vi "Input 信息检测.vi"(9 "Input 配置信息":string[][](table)=[["名称", "点位", "索引号", "逻辑取反"], ["启动按钮", "X100", "0", "0"], ["复位按钮", "X101", "1", "0"], ["暂停按钮", "X102", "2", "0"], ["操作侧安全光栅", "X103", "3", "0"], ["后侧安全光栅", "X104", "4", "0"], ["上层真空检知", "X105", "5", "0"], ["下层真空检知", "X106", "6", "0"], ["上层感应sensor", "X107", "7", "0"], ["下层感应sensor", "X110", "8", "0"], ["传送抓手气缸前位", "X111", "9", "0"], ["传送抓手气缸后位", "X112", "10", "0"], ["上层产品定位气缸前位", "X113", "11", "0"], ["上层产品定位气缸后位", "X114", "12", "0"], ["下层产品定位气缸前位", "X115", "13", "0"], ["下层产品定位气缸后位", "X116", "14", "0"], ["抓手感应产品sensor", "X117", "15", "0"], ["起子1真空检知", "X120", "16", "0"], ["起子2真空检知", "X121", "17", "0"], ["起子3真空检知", "X122", "18", "0"], ["起子4真空检知", "X123", "19", "0"], ["feed01感应sensor", "X124", "20", "0"], ["feed02感应sensor", "X125", "21", "0"], ["feed03感应sensor", "X126", "22", "0"], ["feed04感应sensor", "X127", "23", "0"], ["动子1和2统一坐标sensor", "X130", "24", "0"], ["动子3和4统一坐标sensor", "X131", "25", "0"], ["前后侧统一坐标sensor", "X132", "26", "0"], ["上站允许取料信号", "X133", "27", "0"], ["下站允许投料信号", "X134", "28", "0"], ["上站请求信号", "X135", "29", "0"], ["下站答复信号", "X136", "30", "0"]], 11 "输入":T1) -> (2 "Input  ERROR":string[](array[string]))   [LabVIEW 2017]
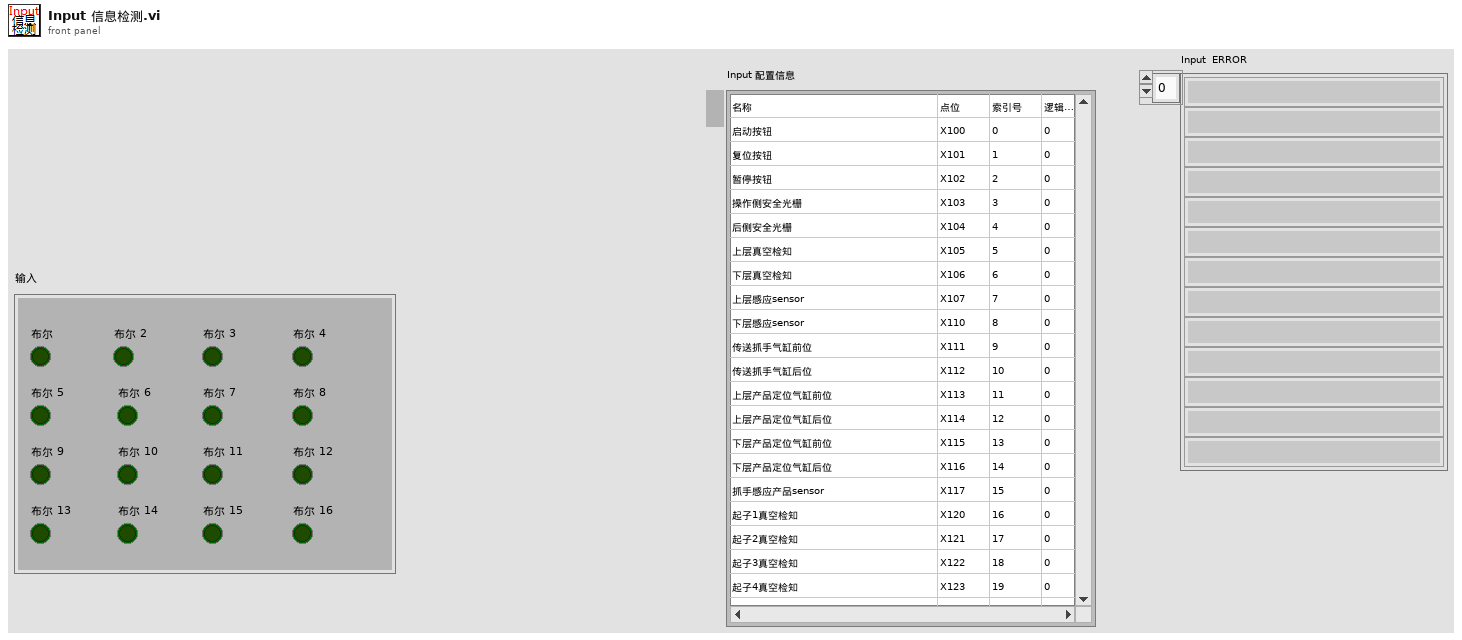
[diagram p1: front panel]
types:
  T1 = typedef "input控件.ctl" = cluster{"布尔":bool, "布尔 2":bool, "布尔 3":bool, "布尔 4":bool, "布尔 5":bool, "布尔 6":bool, "布尔 7":bool, "布尔 8":bool, "布尔 9":bool, "布尔 10":bool, "布尔 11":bool, "布尔 12":bool, "布尔 13":bool, "布尔 14":bool, "布尔 15":bool, "布尔 16":bool}
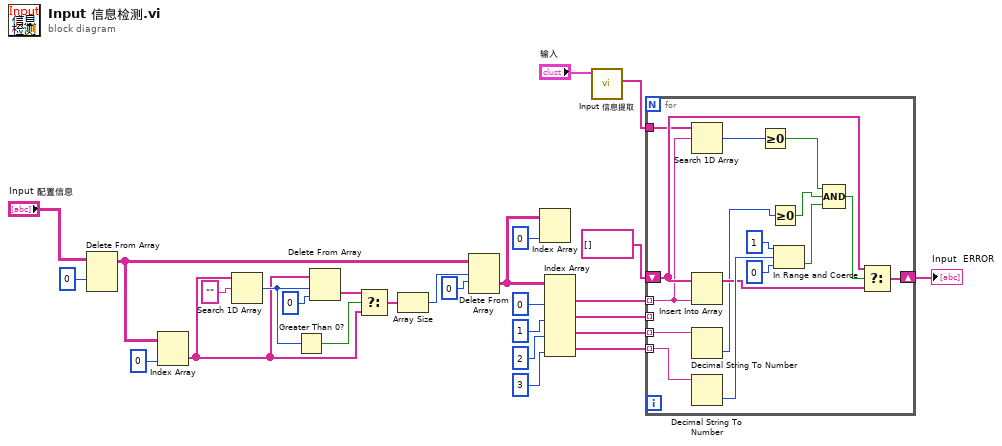
[diagram p0: block diagram]
diagram:
  n1 = Delete From Array(array="Input 配置信息", index (row)=0 ("索引 (行)")) -> (array with subset deleted=w13:string[][])  [unwired: 2 in, 1 out]
  n2 = Index Array(array=w13, index (col)=0 ("禁用的索引 (列)")) -> (element=w16:string[])  [unwired: 1 in]
  n3 = Search 1D Array(1D array=w16, element="") -> (index of element=w20:i32)  [unwired: 1 in]
  n4 = Greater Than 0?(x=w20) -> (x > 0?=w21:bool)
  n5 = Delete From Array(array=w16, length=w20, index=0 ("索引")) -> (deleted portion=w18:string[])  [unwired: 1 out]
  n6 = Select(t=w18, s=w21, f=w16) -> (s? t:f=w15:string[])
  n7 = Array Size(array=w15) -> (size(s)=w17:i32)
  n8 = Delete From Array(array=w13, length=w17, index (row)=0 ("索引 (行)")) -> (deleted portion=w2:string[][])  [unwired: 1 in, 1 out]
  n9 = Index Array(array=w2, index (col)=0 ("禁用的索引 (列)")) -> ()  [unwired: 1 in, 1 out]
  n10 = Index Array(array=w2, index (col) #1=0 ("禁用的索引 (列)"), index (col) #2=1 ("禁用的索引 (列)"), index (col) #3=2 ("禁用的索引 (列)"), index (col) #4=3 ("禁用的索引 (列)")) -> (element #1=w8:string[], element #2=w7:string[], element #3=w6:string[], element #4=w5:string[])  [unwired: 4 in]
  n11 = call "Input 信息提取.vi"("输入"="输入") -> ("输入读取信号"=w3:string[])  [unwired: 10 in]
  n12 = for {
    tunnel: w8 -> [w30] mode=indexing
    tunnel: w7 -> [_] mode=indexing
    tunnel: w6 -> [w42] mode=indexing
    tunnel: w5 -> [w41] mode=indexing
    shift-right: [w32] -> w1
    shift-left: string[] [] -> [w34]
    tunnel: w3 -> [w31]
    n13 = Search 1D Array(1D array=w31, element=w30) -> (index of element=w43:i32)  [unwired: 1 in]
    n14 = Insert Into Array(array=w34, new element=w30) -> (w33:string[])  [unwired: 1 in]
    n15 = Decimal String To Number(string=w42) -> (number=w29:i32)  [unwired: 2 in, 1 out]
    n16 = Decimal String To Number(string=w41) -> (number=w40:i32)  [unwired: 2 in, 1 out]
    n17 = Greater Or Equal To 0?(x=w43) -> (x >= 0?=w37:bool)
    n18 = Greater Or Equal To 0?(x=w29) -> (x >= 0?=w28:bool)
    n19 = In Range and Coerce(upper limit=1 ("下限"), x=w40, lower limit=0 ("下限")) -> (In Range?=w36:bool)  [unwired: 1 out]
    n20 = Compound Arithmetic op=AND(w37, w28, w36) -> (w35:bool)
    n21 = Select(t=w34, s=w35, f=w33) -> (s? t:f=w32:string[])
  }
  "Input  ERROR" <- w1
